vi "Material-ConfigDialog-UI.vi"(11 "error in":errorcluster) -> (15 "error out":errorcluster)   [LabVIEW 2013, in "Material-ConfigDialog.lvclass"]
uses:
  Material-ConfigDialog.lvclass
  Reuse Library/featherweight/Core/Sequencer/FTW-Sequencer.lvclass/FTW-Sequencer.ctl
  Material-ConfigDialog-Page.ctl
  Reuse Library/featherweight/Core/Messaging/Messenger.Actor/FTW-Messenger-Actor.lvclass
  <instrlib>/Keyence LK-G5000/Public/Constant/Comm Interface.ctl
  Glue/Material-Glue-TreeItem.ctl
  Reuse Library/featherweight/Core/Regex/FTW-Regex.vi
  Reuse Library/featherweight/Core/Error/FTW-ERR-StatusException.vi
  Reuse Library/featherweight/Core/Error/FTW-ERR-Clear.vi
  Reuse Library/featherweight/Core/Error/FTW-ERR-ThrowError.vi
  Deploy Application/Material-Application-Constants.vi
  Reuse Library/featherweight/Core/Sequencer/FTW-Sequencer.lvclass
  Reuse Library/featherweight/Core/Messaging/Message.Actor/FTW-Message-Actor.lvclass
  Automation/Material-Automation-Website.ctl
  <instrlib>/Keyence LK-G5000/Keyence LK-G5000.lvlib
panel:
  in  "UI_Tree_Navigation":string(tree) caption="Navigation Tree"
  in  "Hidden Controls\n(Tab Control Container)":enum32{"Just some hidden controls"}(tab)
  out "Status Bar Messages":string
  in  "UI-Button-Save":bool caption="Save Button"
  in  "UI-Button-Cancel":bool caption="Cancel Button"
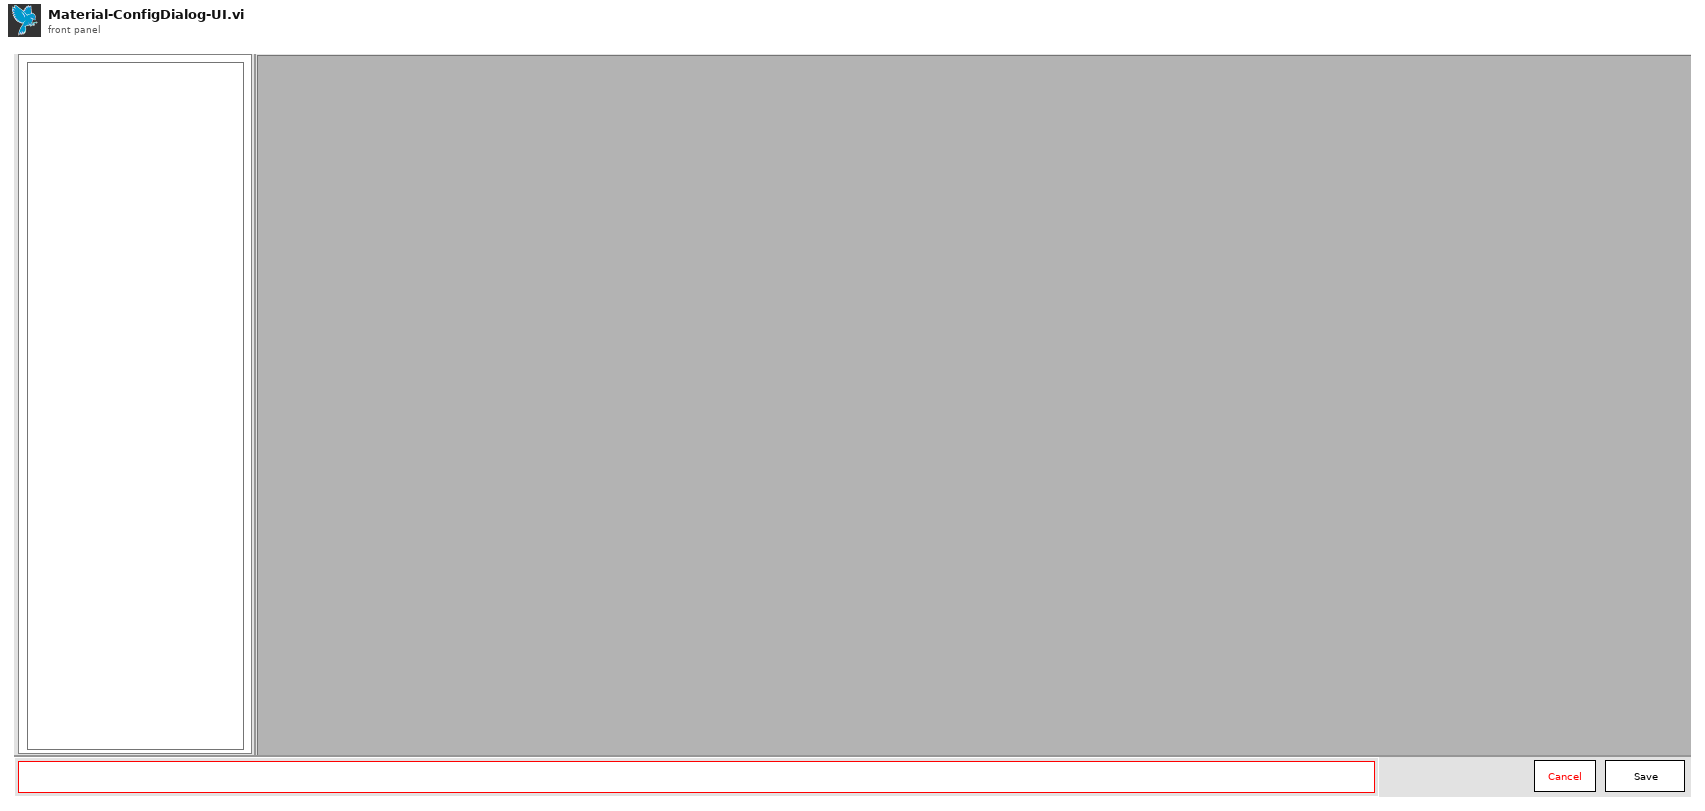
[diagram p1: front panel]
types:
  T1 = typedef "Material-Automation-Website.ctl" = enum16{"Wirebird Labs Home", "Wirebird Labs Support Home", "Wirebird Labs Licensing", "Wirebird Labs Idea Exchange", "Wirebird Labs Report a Bug", "Wirebird Labs Services Status", "Contact Wirebird Labs", "Deploy Documentation", "Deploy Credits", "Deploy Marketing", "Deploy Feature Matrix", "Deploy Purchase", "Deploy Deployment Servers"}
  T2 = typedef "Keyence LK-G5000.lvlib/Comm Interface.ctl" = enum8{"USB", "ETHERNET"}
  T3 = typedef "Material-Glue-TreeItem.ctl" = cluster{"Tag":string, "Parent":string, "Add to Top of Parent":bool, "Type":string, "Indent":i32, "Child Only":bool, "First Cell":string, "Next Cells":string[]}
  T4 = typedef "Material-ConfigDialog.lvclass/Material-ConfigDialog-Page.ctl" = cluster{"Initialized?":bool, "PageID":string, "Messenger":refnum<class "FTW-Messenger-Actor.lvclass">}
  T5 = cluster{"Configuration Dialog Mailbox":refnum<event-registration>}
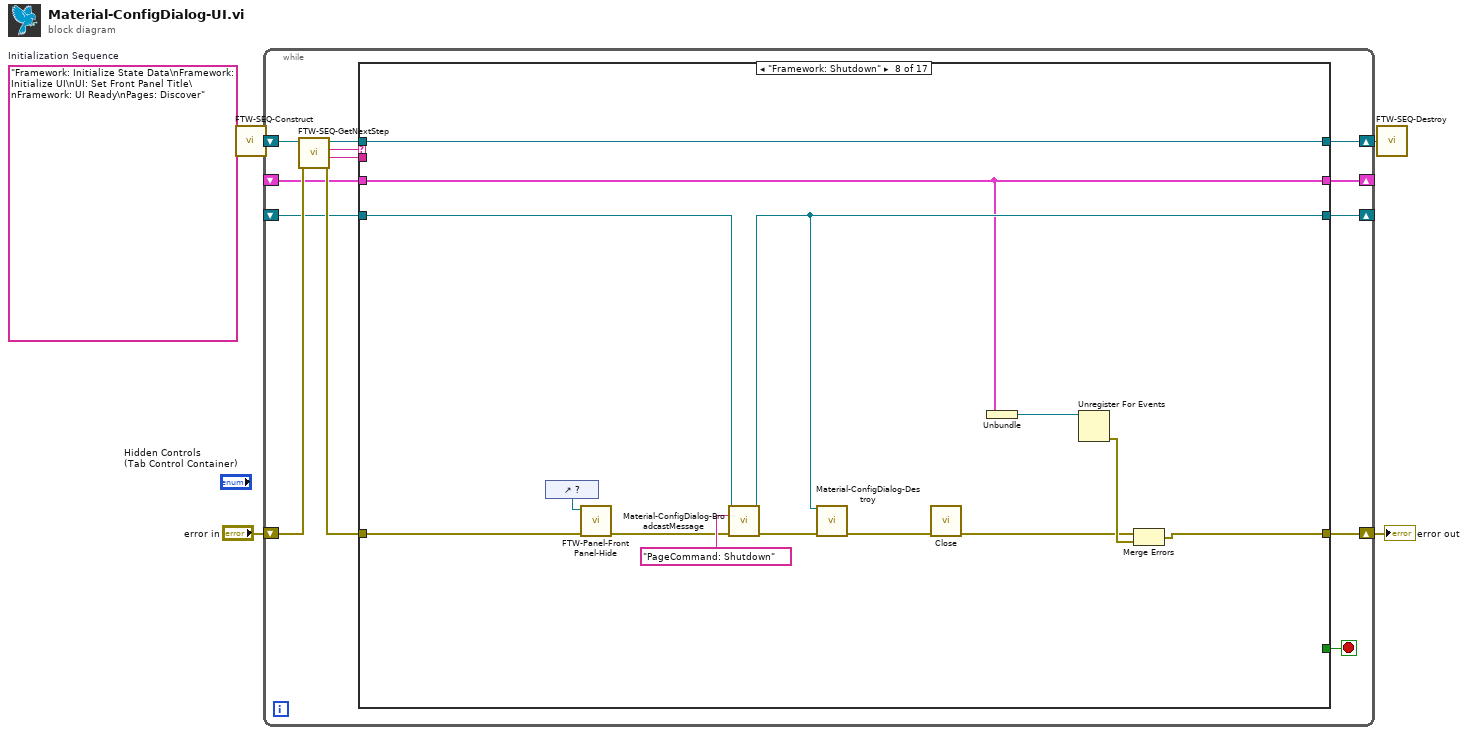
[diagram p0: block diagram]
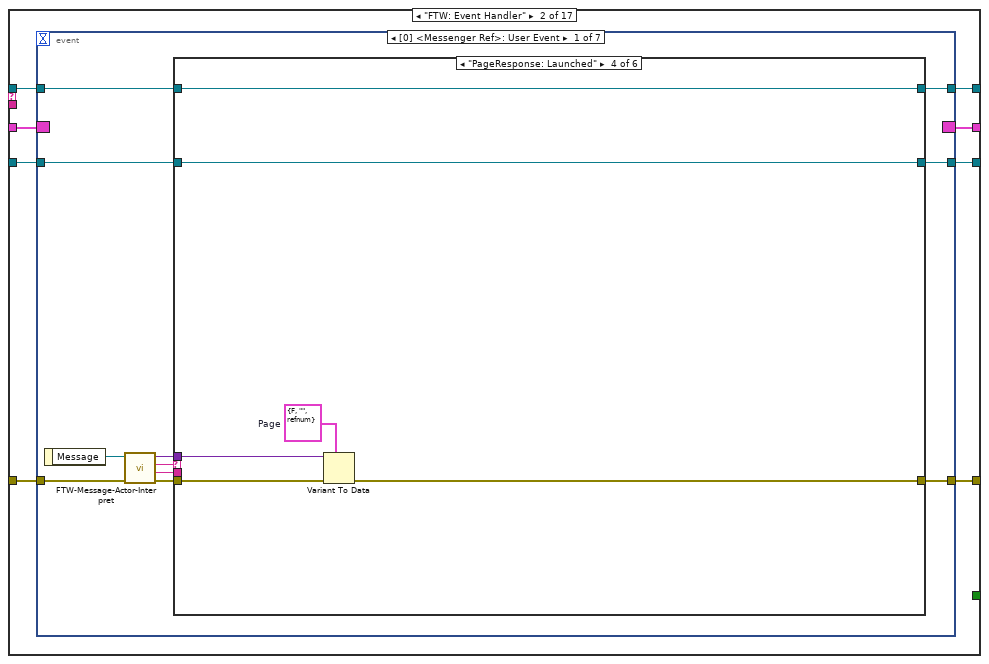
[diagram p3: hidden frame]
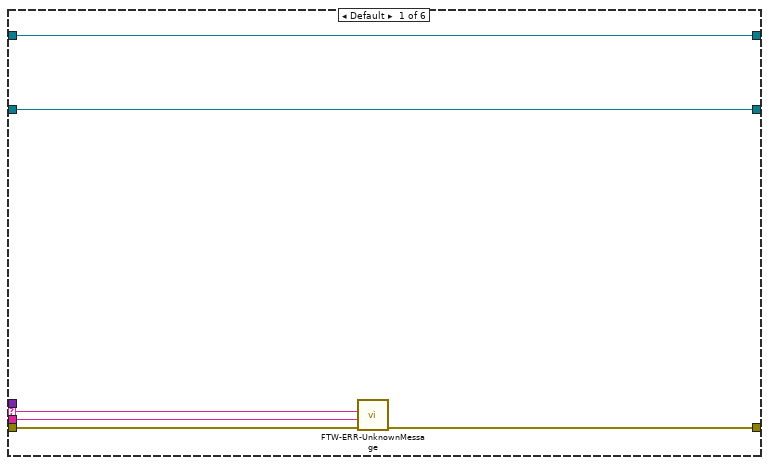
[diagram p4: hidden frame]
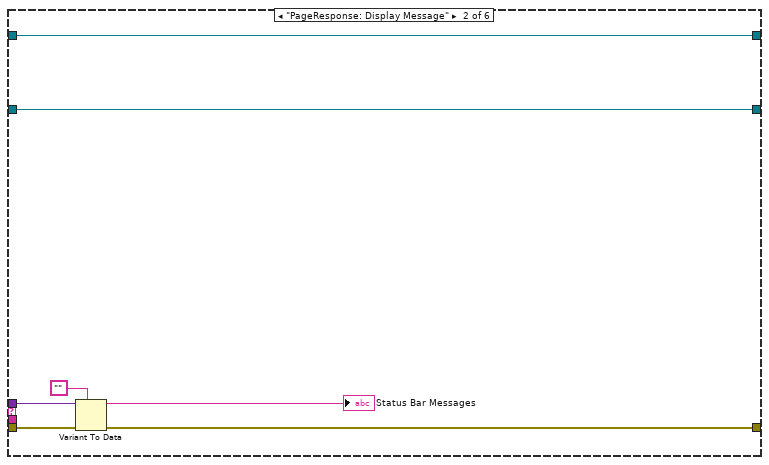
[diagram p5: hidden frame]
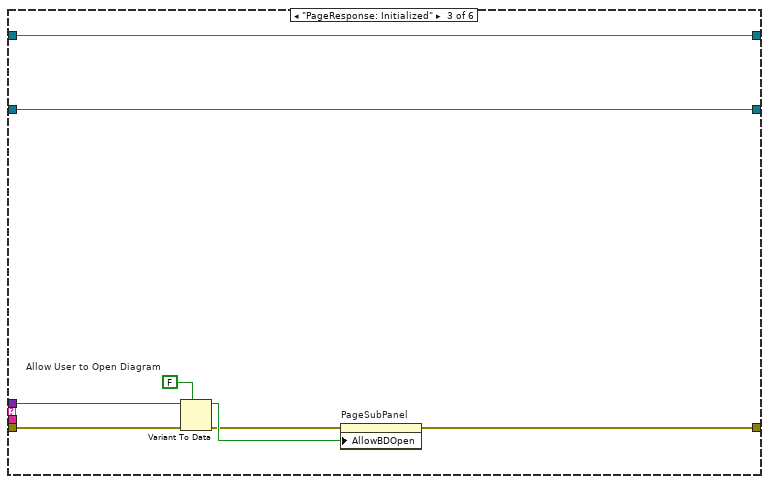
[diagram p6: hidden frame]
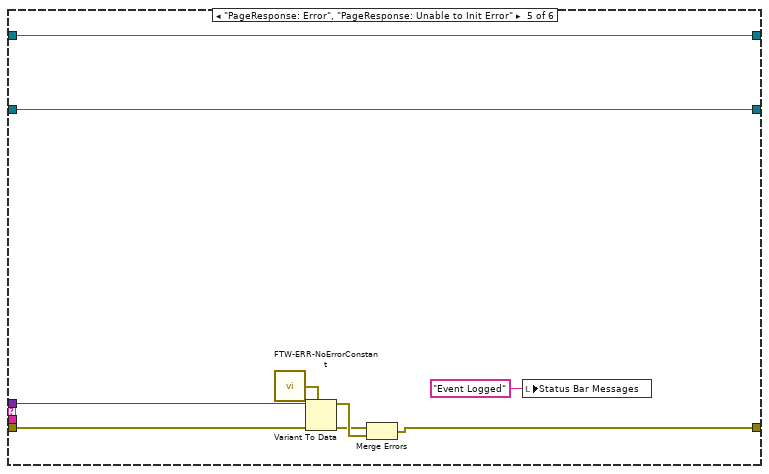
[diagram p7: hidden frame]
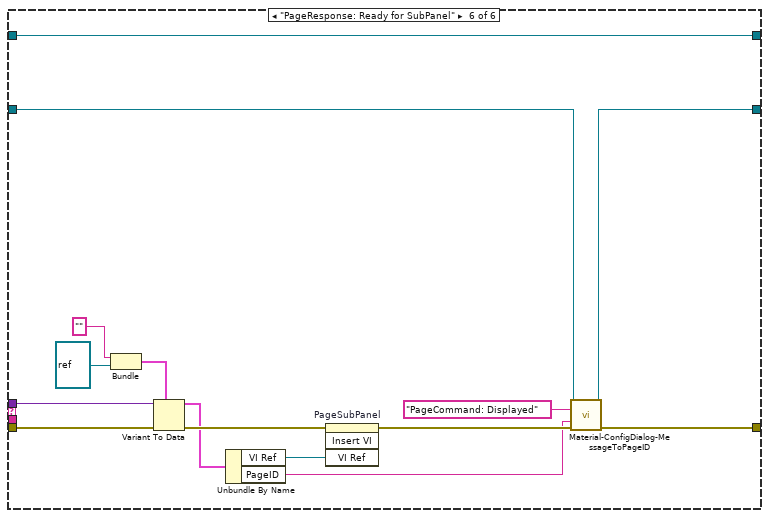
[diagram p8: hidden frame]
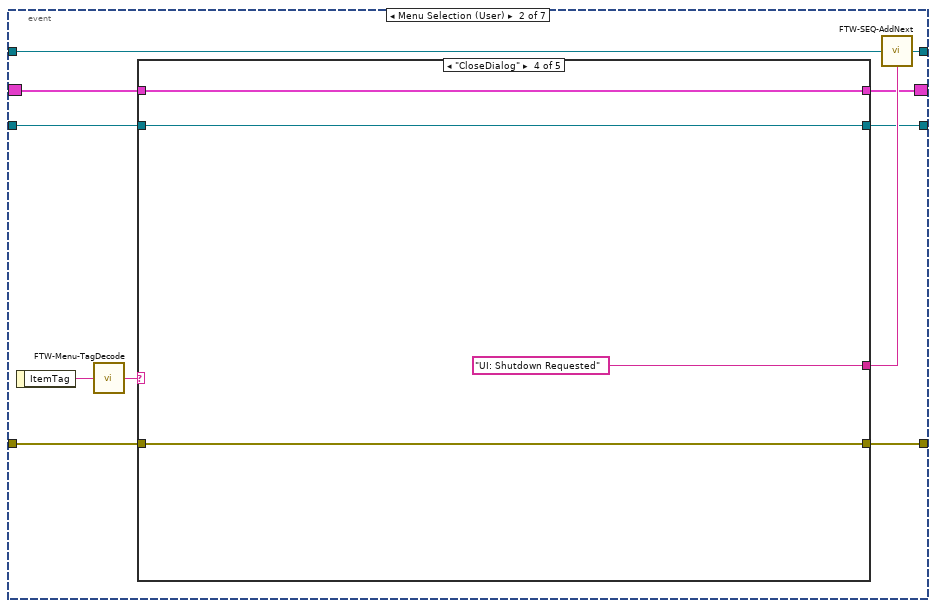
[diagram p9: hidden frame]
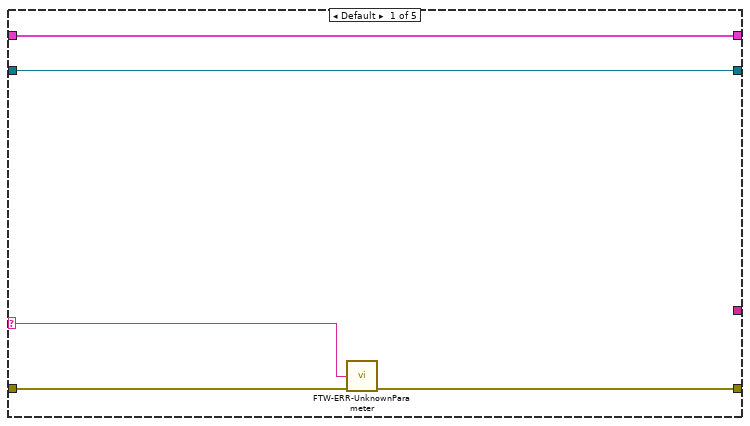
[diagram p10: hidden frame]
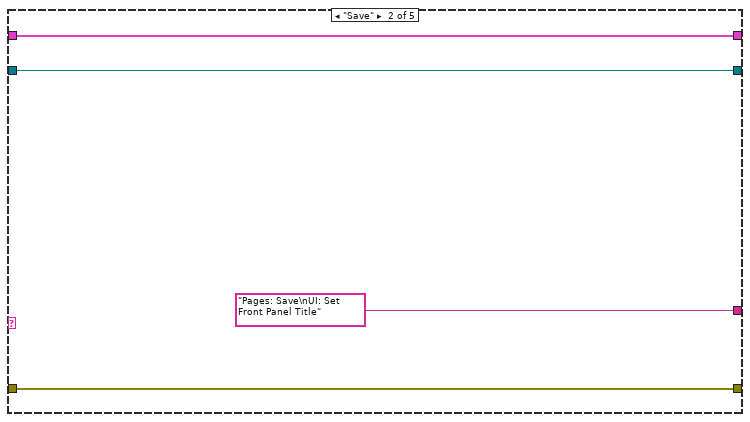
[diagram p11: hidden frame]
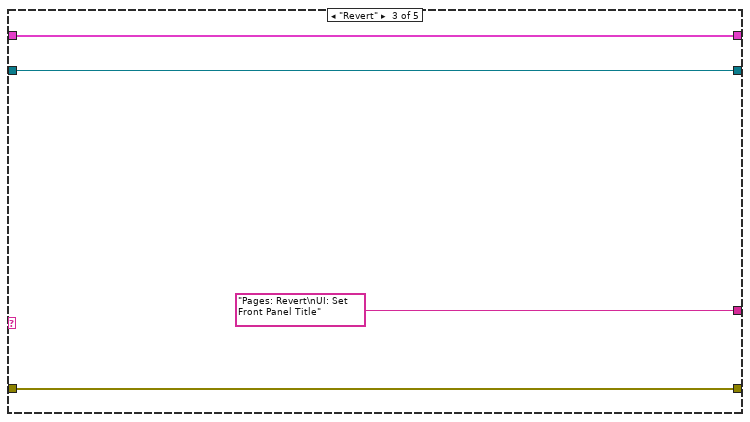
[diagram p12: hidden frame]
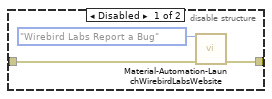
[diagram p14: hidden frame]
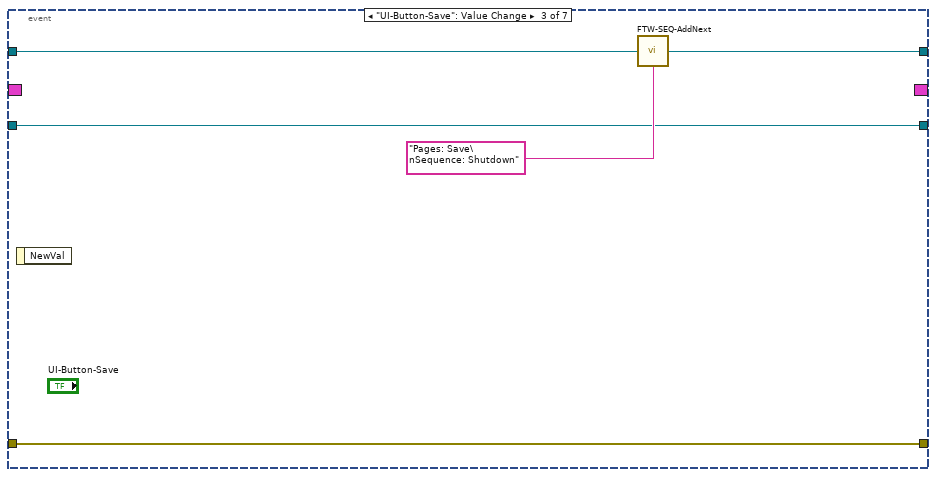
[diagram p15: hidden frame]
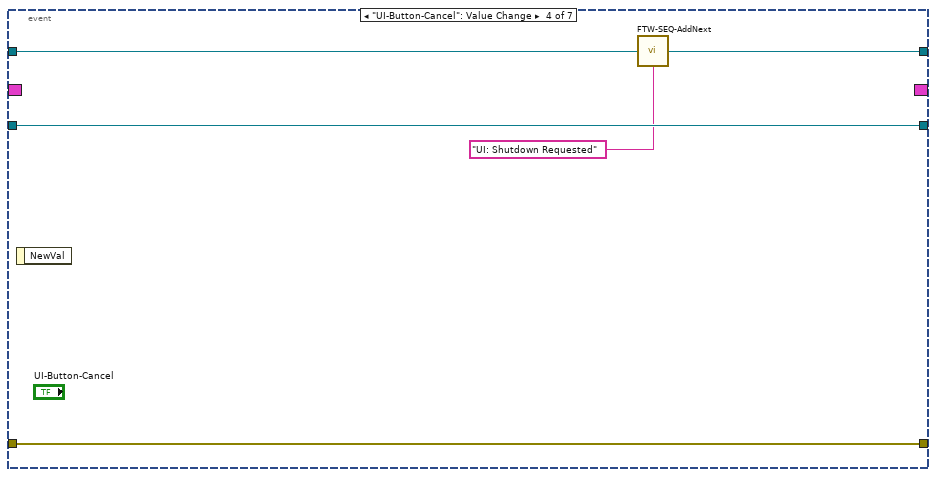
[diagram p16: hidden frame]
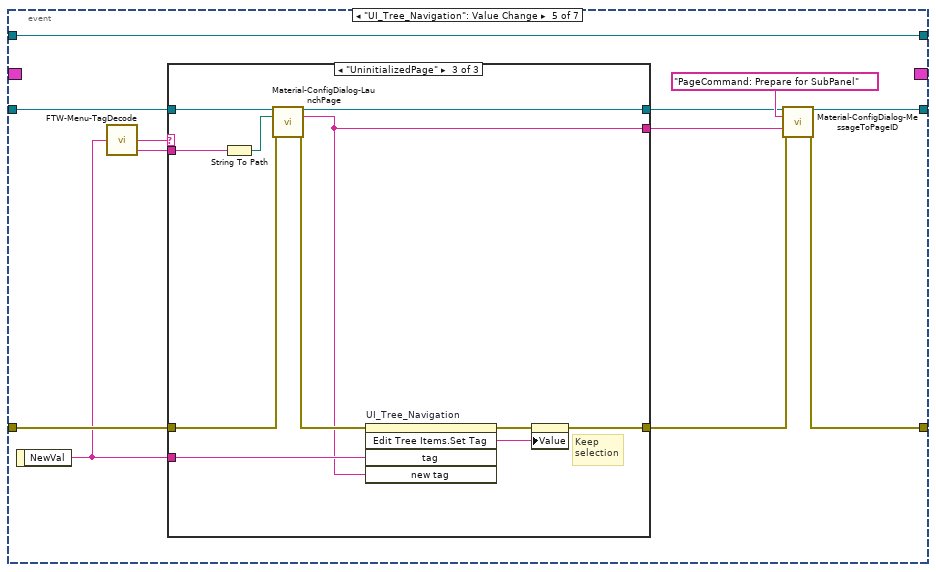
[diagram p17: hidden frame]
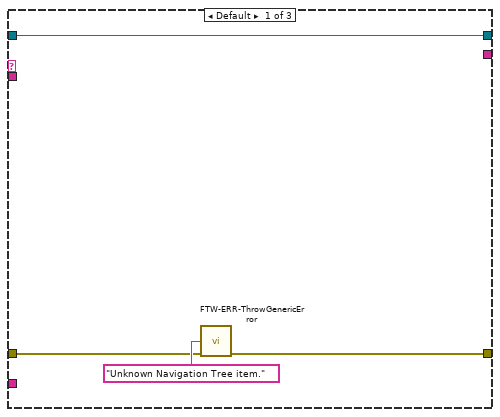
[diagram p18: hidden frame]
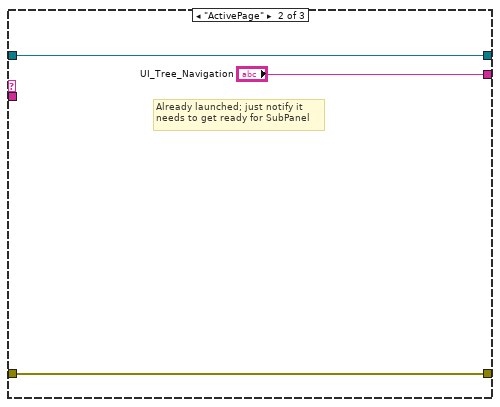
[diagram p19: hidden frame]
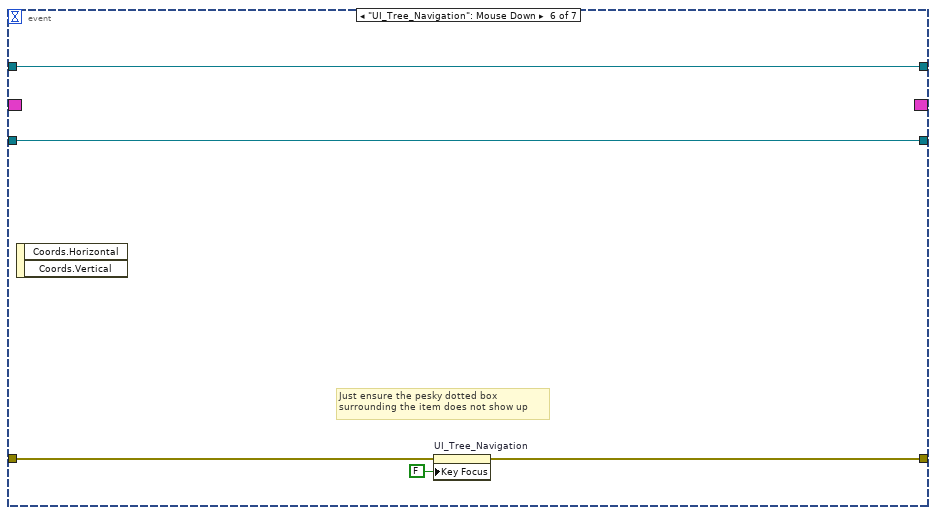
[diagram p20: hidden frame]
diagram:
  w5 = "Framework: Initialize State Data\nFramework: Initialize UI\nUI: Set Front Panel Title\nFramework: UI Ready\nPages: Discover"  # Initialization Sequence
  n1 = call "FTW-SEQ-Construct.vi"("Initial Sequence"=w5) -> ("Sequencer"=w2:refnum<class "FTW-Sequencer.lvclass">)
  n2 = while {
    shift-right: [w16] -> w1
    shift-left: w2 -> [w7]
    shift-right: [w17] -> w4
    shift-left: "error in" -> [w15]
    shift-right: [w10] -> _
    shift-left: _ -> [w11]
    shift-right: [w9] -> _
    shift-left: _ -> [w8]
    stop <- w12 stop-if-true
    n3 = call "FTW-SEQ-GetNextStep.vi"("error in"=w15, "Sequencer"=w7) -> ("error out"=w18:errorcluster, "Job Data"=w6:string, "Current Job"=w13:string, "Sequencer out"=w14:refnum<class "FTW-Sequencer.lvclass">)  [unwired: 6 in]
    n4 = case shown="\"Framework: Shutdown\"" w13 {
      selector: w13 -> [_ _ _ _ _ _ w234 _ _ _ _ _ _ _ _ _ _]
      tunnel: [w20 w28 w180 w198 w223 w229 w236 w253 w254 w262 w268 w273 w275 w291 w312 w325 w334] -> w17
      tunnel: w18 -> [w20 w27 w185 w199 w224 w230 w237 w246 w255 w262 w268 w273 w275 w291 w300 w321 w329]
      tunnel: w14 -> [w22 w30 w184 w221 w227 w233 w239 w251 w260 w264 w265 w272 w279 w293 w315 w328 w336]
      tunnel: [w22 w29 w184 w221 w227 w233 w239 w251 w260 w264 w270 w272 w281 w293 w315 w328 w336] -> w16
      tunnel: [_ _ _ _ _ _ _ _ TRUE _ _ _ _ _ _ _ _] -> w12
      tunnel: w11 -> [w21 w25 _ w220 w226 w232 w238 w243 w258 w263 w269 w274 w282 w298 w314 w327 w335]
      tunnel: [w21 w26 w186 w220 w226 w232 w238 w243 w258 w263 w269 w274 w282 w298 w314 w327 w335] -> w10
      tunnel: [w19 w24 w183 w219 w225 w231 w235 w247 w257 w261 w266 w271 w280 w294 w301 w326 w333] -> w9
      tunnel: w8 -> [w19 w23 _ w219 w225 w231 w235 w248 w257 w261 w266 w271 w280 w294 w301 w322 w330]
      tunnel: w6 -> [_ _ _ _ _ _ _ _ _ _ _ _ _ _ _ _ _]
      frame "--------- Framework ---------" {
      }
      frame "FTW: Event Handler" {
        n5 = event shown="[0] <Messenger Ref>: User Event" {
          selector: w25 -> [_ w93 _ _ _ _ _]
          dyn-events: [_ w94 _ _ _ _ _] -> w26
          timeout: _ -> [_ _ _ _ _ _ _]
          tunnel: w30 -> [w34 w99 w129 w135 w148 w170 w174]
          tunnel: [w35 w103 w133 w138 w148 w170 w177] -> w29
          tunnel: [w38 w100 w132 w136 w149 w171 w178] -> w28
          tunnel: w27 -> [w39 w101 w132 w136 w145 w172 w178]
          tunnel: [w37 w96 w130 w137 w147 w169 w175] -> w24
          tunnel: w23 -> [w36 w95 w130 w137 w142 w169 w175]
          event User Event {
            n6 = event-data() -> ("Message"=w40:refnum<class "FTW-Message.lvclass">)  [unwired: 1 in]
            n7 = call "FTW-Message-Actor-Interpret.vi"("error in"=w39, "Message"=w40) -> ("error out"=w41:errorcluster, "Sender"=w31:string, "Parameter"=w33:string, "Payload"=w32:variant)  [unwired: 6 in]
            n8 = case shown="\"PageResponse: Launched\"" w33 {
              selector: w33 -> [w43 _ _ _ _ _]
              tunnel: w32 -> [_ w54 w55 w65 w77 w92]
              tunnel: [w46 w52 w56 w63 w69 w85] -> w38
              tunnel: w41 -> [w47 w53 w60 w64 w76 w91]
              tunnel: [w44 w48 w62 w68 w73 w87] -> w37
              tunnel: w36 -> [w44 w48 w62 w68 w73 w88]
              tunnel: [w45 w49 w61 w67 w74 w90] -> w35
              tunnel: w34 -> [w45 w49 w61 w67 w74 w90]
              tunnel: w31 -> [w42 _ _ _ _ _]
              frame Default {
                n9 = call "FTW-ERR-UnknownMessage.vi"("error in"=w47, "Sender"=w42, "Unknown Parameter"=w43) -> ("error out"=w46:errorcluster)  [unwired: 8 in]
              }
              frame "PageResponse: Display Message" {
                n10 = Variant To Data(error in=w53, type="", Variant=w54) -> (data=→"Status Bar Messages":string, error out=w52:errorcluster)
              }
              frame "PageResponse: Initialized" {
                w59 = FALSE  # Allow User to Open Diagram
                n11 = Variant To Data(error in=w60, type=w59, Variant=w55) -> (data=w58:bool, error out=w57:errorcluster)
                n12 = property on="PageSubPanel" class="SubPnl"(error in=w57, "AllowBDOpen"=w58) -> (error out=w56:errorcluster)  [unwired: 1 in, 1 out]
              }
              frame "PageResponse: Launched" {
                w66 = T4 {"Initialized?"=FALSE, "PageID"="", "Messenger"=refnum}  # Page
                n13 = Variant To Data(error in=w64, type=w66, Variant=w65) -> (error out=w63:errorcluster)  [unwired: 1 out]
              }
              frame "PageResponse: Error", "PageResponse: Unable to Init Error" {
                n14 = call "FTW-ERR-NoErrorConstant.vi"() -> ("no error"=w75:errorcluster)
                n15 = Variant To Data(error in=w76, type=w75, Variant=w77) -> (data=w71:errorcluster, error out=w70:errorcluster)
                n16 = Merge Errors(w70, w71) -> (w69:errorcluster)
                n17 = local write "Status Bar Messages"("Event Logged" ("Status Bar Messages")) -> ()
              }
              frame "PageResponse: Ready for SubPanel" {
                n18 = Bundle("PageID"="", "VI Ref"=refnum<vi> refnum) -> (w81:cluster{"PageID":string, "VI Ref":refnum<vi>})  [unwired: 1 in]
                n19 = Variant To Data(error in=w91, type=w81, Variant=w92) -> (data=w80:cluster{"PageID":string, "VI Ref":refnum<vi>}, error out=w84:errorcluster)
                n20 = Unbundle By Name(w80) -> ("VI Ref"=w79:refnum<vi>, "PageID"=w78:string)
                n21 = invoke on="PageSubPanel" class="SubPanel" method="Insert VI"(error in=w84, "VI Ref"=w79) -> (error out=w86:errorcluster)  [unwired: 2 in, 3 out]
                n22 = call "Material-ConfigDialog-MessageToPageID.vi"("Configuration Dialog"=w88, "Parameter"="PageCommand: Displayed", "PageID"=w78, "error in"=w86) -> ("Configuration Dialog out"=w87:refnum<class "Material-ConfigDialog.lvclass">, "error out"=w85:errorcluster)  [unwired: 10 in]
              }
            }
          }
          event Menu Selection (User) {
            n23 = event-data() -> ("ItemTag"=w98:string)  [unwired: 1 in]
            n24 = call "FTW-Menu-TagDecode.vi"("Menu Item Tag"=w98) -> ("Command"=w97:string)  [unwired: 1 in, 2 out]
            n25 = case shown="\"CloseDialog\"" w97 {
              selector: w97 -> [w105 _ _ _ _]
              tunnel: [_ "Pages: Save\nUI: Set Front Panel Title" ("Add to Top of Queue") "Pages: Revert\nUI: Set Front Panel Title" ("Add to Top of Queue") "UI: Shutdown Requested" ("Add to Top of Queue") _] -> w102
              tunnel: w101 -> [w108 w111 w115 w119 w124]
              tunnel: [w107 w111 w115 w119 w123] -> w100
              tunnel: [w106 w110 w114 w118 w122] -> w96
              tunnel: w95 -> [w106 w110 w114 w118 w122]
              tunnel: [w104 w109 w113 w117 w121] -> w94
              tunnel: w93 -> [w104 w109 w113 w117 w121]
              frame Default {
                n26 = call "FTW-ERR-UnknownParameter.vi"("Unknown Parameter"=w105, "error in"=w108) -> ("error out"=w107:errorcluster)  [unwired: 13 in]
              }
              frame "Save" {
              }
              frame "Revert" {
              }
              frame "CloseDialog" {
              }
              frame "ReportBug" {
                n27 = disable-structure shown="Enabled" {
                  disable-tunnel: w124 -> [w127 w128]
                  disable-tunnel: [w126 w128] -> w123
                  frame Disabled {
                    n28 = call "Material-Automation-LaunchWirebirdLabsWebsite.vi"("Site to Launch"=Material-Automation-Website."Wirebird Labs Report a Bug", "error in"=w127) -> ("error out"=w126:errorcluster)  [unwired: 13 in]
                  }
                  frame Enabled {
                  }
                }
              }
            }
            n29 = call "FTW-SEQ-AddNext.vi"("Add Next in Sequence"=w102, "Sequencer"=w99) -> ("Sequencer out"=w103:refnum<class "FTW-Sequencer.lvclass">)  [unwired: 2 in]
          }
          event "UI-Button-Save": Value Change {
            n30 = event-data() -> ()  [unwired: 1 in, 1 out]
            n31 = call "FTW-SEQ-AddNext.vi"("Add Next in Sequence"="Pages: Save\nSequence: Shutdown" ("Add to Top of Queue"), "Sequencer"=w129) -> ("Sequencer out"=w133:refnum<class "FTW-Sequencer.lvclass">)  [unwired: 2 in]
          }
          event "UI-Button-Cancel": Value Change {
            n32 = event-data() -> ()  [unwired: 1 in, 1 out]
            n33 = call "FTW-SEQ-AddNext.vi"("Add Next in Sequence"="UI: Shutdown Requested" ("Add to Top of Queue"), "Sequencer"=w135) -> ("Sequencer out"=w138:refnum<class "FTW-Sequencer.lvclass">)  [unwired: 2 in]
          }
          event "UI_Tree_Navigation": Value Change {
            n34 = event-data() -> ("NewVal"=w140:string)  [unwired: 1 in]
            n35 = call "FTW-Menu-TagDecode.vi"("Menu Item Tag"=w140) -> ("Command"=w146:string, "Payload"=w143:string)  [unwired: 1 in, 1 out]
            n36 = case shown="\"UninitializedPage\"" w146 {
              tunnel: w145 -> [w153 w157 w168]
              tunnel: [w152 w157 w159] -> w144
              tunnel: w143 -> [_ _ w167]
              tunnel: w142 -> [w151 w156 w165]
              tunnel: [w151 w156 w164] -> w141
              tunnel: w140 -> [_ _ w162]
              tunnel: [_ "UI_Tree_Navigation" w161] -> w139
              frame Default {
                n37 = call "FTW-ERR-ThrowGenericError.vi"("Error Message"="Unknown Navigation Tree item.", "error in"=w153) -> ("error out"=w152:errorcluster)  [unwired: 13 in]
              }
              frame "ActivePage" {
                # "Already launched; just notify it\nneeds to get ready for SubPanel"
              }
              frame "UninitializedPage" {
                # "Keep\nselection"
                n38 = String To Path(string=w167) -> (path=w166:path)
                n39 = call "Material-ConfigDialog-LaunchPage.vi"("Configuration Dialog"=w165, "Configuration Page VI Filepath"=w166, "error in"=w168) -> ("Configuration Dialog out"=w164:refnum<class "Material-ConfigDialog.lvclass">, "New Navigation Tree Tag"=w161:string, "error out"=w163:errorcluster)  [unwired: 9 in, 1 out]
                n40 = invoke on="UI_Tree_Navigation" class="Tree (strict)" method="Edit Tree Items.Set Tag"(error in=w163, "tag"=w162, "new tag"=w161) -> (error out=w160:errorcluster, "Edit Tree Items:Set Tag"=w158:string)  [unwired: 2 in, 3 out]
                n41 = property on="UI_Tree_Navigation" class="Tree (strict)"(error in=w160, "Value"=w158) -> (error out=w159:errorcluster)  [unwired: 1 in, 1 out]
              }
            }
            n42 = call "Material-ConfigDialog-MessageToPageID.vi"("Configuration Dialog"=w141, "Parameter"="PageCommand: Prepare for SubPanel", "PageID"=w139, "error in"=w144) -> ("Configuration Dialog out"=w147:refnum<class "Material-ConfigDialog.lvclass">, "error out"=w149:errorcluster)  [unwired: 10 in]
          }
          event "UI_Tree_Navigation": Mouse Down {
            # "Just ensure the pesky dotted box\nsurrounding the item does not show up"
            n43 = event-data() -> ()  [unwired: 1 in, 2 out]
            n44 = property on="UI_Tree_Navigation" class="Tree (strict)"(error in=w172, "Key Focus"=FALSE) -> (error out=w171:errorcluster)  [unwired: 1 in, 1 out]
          }
          event Panel Close? {
            n45 = event-data() -> ()  [unwired: 1 in, 1 out]
            n46 = call "FTW-SEQ-AddNext.vi"("Add Next in Sequence"="UI: Shutdown Requested" ("Add to Top of Queue"), "Sequencer"=w174) -> ("Sequencer out"=w177:refnum<class "FTW-Sequencer.lvclass">)  [unwired: 2 in]
            n47 = event-data("Discard?"=TRUE) -> ()  [unwired: 1 in, 1 out]
          }
        }
      }
      frame "Framework: Initialize State Data" {
        n48 = call "Material-ConfigDialog-Construct.vi"("error in"=w185) -> ("Configuration Dialog"=w183:refnum<class "Material-ConfigDialog.lvclass">, "Configuration Dialog Mailbox"=w187:refnum<event-registration>, "error out"=w181:errorcluster)  [unwired: 12 in]
        n49 = call <instrlib>:"Initialize.vi"("error in (no error)"=w181, "Comm Interface"=Comm_Interface."USB") -> ("error out"=w180:errorcluster)  [unwired: 9 in]
        n50 = Bundle("Configuration Dialog Mailbox"=w187) -> (w186:T5)  [unwired: 1 in]
      }
      frame "Framework: Initialize UI" {
        w195 = cluster{"Height":i16, "Width":i16} {"Height"=2, "Width"=2}  # Breathing Room
        w201 = i16 40 ("Vertical")
        w204 = i16 240 ("Horizontal")
        w211 = 2000  # Much wider than ever expected to be
        n51 = invoke on="UI_Tree_Navigation" class="Tree (strict)" method="Edit Tree Items.Delete"("Delete Children"=TRUE ("Delete Children?")) -> (error out=w193:errorcluster)  [unwired: 4 in, 4 out]
        n52 = call "Material-Application-MinimumPageSize.vi"("error in"=w199) -> ("Minimum Pane Size"=w192:cluster{"Horizontal":i16, "Vertical":i16}, "error out"=w210:errorcluster)  [unwired: 13 in]
        n53 = Bundle By Name(cluster=w192, "Horizontal"=w204) -> (w209:cluster{"Horizontal":i16, "Vertical":i16})
        n54 = Bundle By Name(cluster=w192, "Horizontal"=i16 310, "Vertical"=w201) -> (w208:cluster{"Horizontal":i16, "Vertical":i16})
        n55 = global read "Material-Application-Constants.vi" "Color.Selection"() -> (w189:u32)
        n56 = Add(x=cluster{"Horizontal":i16, "Vertical":i16} {"Horizontal"=24, "Vertical"=0}, y=w192) -> (x+y=w190:cluster{"Horizontal":i16, "Vertical":i16})
        n57 = Unbundle By Name(w190) -> ("Horizontal"=w205:i16, "Vertical"=w202:i16)
        n58 = property on="UserInterface-Pane-Page" class="Pane"(error in=w210, "Minimum Pane Size"=w190) -> (error out=w217:errorcluster)  [unwired: 1 in, 1 out]
        n59 = property on="UserInterface-Pane-Navigation" class="Pane"("Minimum Pane Size"=w209) -> (error out=w215:errorcluster)  [unwired: 2 in, 1 out]
        n60 = property on="UserInterface-Pane-Buttons" class="Pane"("Minimum Pane Size"=w208) -> (error out=w214:errorcluster)  [unwired: 2 in, 1 out]
        n61 = property on="UI_Tree_Navigation" class="Tree (strict)"(error in=w193, "Value"="", "SelMode"=1 ("Selection Mode"), "ActiveColNum"=0 ("Active Cell:Active Column Number"), "Width"=w211, "SelColor"=w189) -> (error out=w188:errorcluster)  [unwired: 1 in, 1 out]
        n62 = Add(x=w204, y=w205) -> (x+y=w203:i16)
        n63 = Add(x=w201, y=w202) -> (x+y=w200:i16)
        n64 = Bundle By Name(cluster=cluster{"Height":i16, "Width":i16} {"Height"=0, "Width"=0} ("Size"), "Height"=w200, "Width"=w203) -> (w206:cluster{"Height":i16, "Width":i16})
        n65 = Merge Errors(w188, w217, w215, w214) -> (w216:errorcluster)
        n66 = Add(x=w195, y=w206) -> (x+y=w196:cluster{"Height":i16, "Width":i16})
        n67 = invoke class="VI" method="FP.Run-Time Position.Centered"(error in=w216, "Monitor"=w196) -> (error out=w198:errorcluster)  [unwired: 3 in, 4 out]
      }
      frame "Framework: UI Ready" {
        n68 = control-ref of="?"() -> (w222:refnum<vi>)
        n69 = call "FTW-Panel-FrontPanel-Open.vi"("error in"=w224, "VI Ref"=w222) -> ("error out"=w223:errorcluster)  [unwired: 8 in, 1 out]
      }
      frame "FTW: Error Handler" {
        n70 = call "FTW-ERR-SerializeForLog.vi"("error in"=w230) -> ("Serialized Error"=w228:string)
        n71 = local write "Status Bar Messages"(w228) -> ()
        n72 = call "FTW-ERR-NoErrorConstant.vi"() -> ("no error"=w229:errorcluster)
      }
      frame "FTW: Unknown Job", Default {
        n73 = call "FTW-ERR-UnknownJob.vi"("error in"=w237, "Unknown Job"=w234) -> ("error out"=w236:errorcluster)  [unwired: 9 in]
      }
      frame "Framework: Shutdown" {
        n74 = control-ref of="?"() -> (w244:refnum<vi>)
        n75 = call "FTW-Panel-FrontPanel-Hide.vi"("error in"=w246, "VI Ref"=w244) -> ("error out"=w245:errorcluster)  [unwired: 8 in, 1 out]
        n76 = call "Material-ConfigDialog-BroadcastMessage.vi"("Configuration Dialog"=w248, "Parameter"="PageCommand: Shutdown", "error in"=w245) -> ("Configuration Dialog out"=w247:refnum<class "Material-ConfigDialog.lvclass">, "error out"=w249:errorcluster)  [unwired: 11 in]
        n77 = call "Material-ConfigDialog-Destroy.vi"("Configuration Dialog"=w247, "error in"=w249) -> ("error out"=w241:errorcluster)  [unwired: 13 in]
        n78 = call <instrlib>:"Close.vi"("error in (no error)"=w241) -> ("error out"=w240:errorcluster)  [unwired: 10 in]
        n79 = Unbundle(w243) -> ("Configuration Dialog Mailbox"=w242:refnum<event-registration>)
        n80 = Unregister For Events(event registration refnum=w242) -> (error out=w252:errorcluster)  [unwired: 1 in]
        n81 = Merge Errors(w240, w252) -> (w253:errorcluster)
      }
      frame "Framework: Exit" {
        n82 = control-ref of="?"() -> (w256:refnum<vi>)
        n83 = call "FTW-Panel-FrontPanel-Close.vi"("error in"=w255, "VI Ref"=w256) -> ("error out"=w254:errorcluster)  [unwired: 8 in, 1 out]
      }
      frame "--------- Sequences ---------" {
      }
      frame "Sequence: Shutdown" {
        w267 = "Framework: Shutdown\nFramework: Exit"  # Application Shutdown
        n84 = call "FTW-SEQ-AddNext.vi"("Add Next in Sequence"=w267, "Sequencer"=w265) -> ("Sequencer out"=w270:refnum<class "FTW-Sequencer.lvclass">)  [unwired: 2 in]
      }
      frame "--------- Application Logic ---------" {
      }
      frame "UI: Shutdown Requested" {
        w276 = TRUE  # Shutdown Conditionally Allowed?
        n85 = case shown="True" w276 {
          tunnel: [w283 w287] -> w278
          tunnel: "Sequence: Shutdown" ("Add to Top of Queue") -> [w283 w285]
          frame False {
          }
          frame True {
            w286 = ""  # Do nothing... return to dialog without shutting down.
            n86 = Two Button Dialog(message="Are you sure you want to shut down?", 1:"Shutdown now" ("F button name (\"Cancel\")"), 2:"Not yet" ("T button name (\"OK\")")) -> (T button?=w288:bool)
            n87 = Select(t=w286, s=w288, f=w285) -> (s? t:f=w287:string)
          }
        }
        n88 = call "FTW-SEQ-AddNext.vi"("Add Next in Sequence"=w278, "Sequencer"=w279) -> ("Sequencer out"=w281:refnum<class "FTW-Sequencer.lvclass">)  [unwired: 2 in]
      }
      frame "UI: Set Front Panel Title" {
        w292 = FALSE  # Show Dirty Dot?
        n89 = Select(t="Deployment Configuration*", s=w292, f="Deployment Configuration") -> (s? t:f=w297:string)
        n90 = property class="VI"("Front Panel.Title"=w297) -> ()  [unwired: 2 in, 2 out]
      }
      frame "Pages: Discover" {
        w305 = FALSE  # Collapse all new items?
        w308 = TRUE  # Delete Tree Items First?
        # "Make it go to the default page; in the future,\nthis can be replaced by a \"Last Page Visited\""
        n91 = call "Material-ConfigDialog-DiscoverPages.vi"("Custom Config Pages Directory"=path "", "error in"=w300) -> ("Display Names"=w303:string[], "Tree Tags"=w304:string[], "error out"=w302:errorcluster)  [unwired: 9 in, 2 out]
        n92 = for {
          tunnel: T3 {"Tag"="", "Parent"="", "Add to Top of Parent"=FALSE, "Type"="", "Indent"=0, "Child Only"=FALSE, "First Cell"="", "Next Cells"=[]} -> [w320]
          tunnel: [w319] -> w306 mode=indexing
          tunnel: w304 -> [w316] mode=indexing
          tunnel: w303 -> [w318] mode=indexing
          n93 = Bundle By Name(cluster=w320, "Child Only"=TRUE, "First Cell"=w318, "Tag"=w316) -> (w319:T3)
        }
        n94 = control-ref of="UI_Tree_Navigation"() -> (w310:refnum<vi>)
        n95 = call "Material-Glue-Tree-AddItems.vi"("Tree Ctl Ref"=w310, "Tree Items to Create"=w306, "Delete Tree Items First?"=w308, "Collapse all new items?"=w305, "error in"=w302) -> ("error out"=w309:errorcluster)  [unwired: 8 in, 2 out]
        n96 = Index Array(array=w304, index=0) -> (element=w311:string)
        n97 = property on="UI_Tree_Navigation" class="Tree (strict)"(error in=w309, "Val(Sgnl)"=w311) -> (error out=w312:errorcluster)  [unwired: 1 in, 1 out]
      }
      frame "Pages: Save" {
        n98 = local read "UI_Tree_Navigation"() -> (w324:string)
        n99 = call "Material-ConfigDialog-MessageToPageID.vi"("Configuration Dialog"=w322, "Parameter"="PageCommand: Settings Saved", "PageID"=w324, "error in"=w321) -> ("Configuration Dialog out"=w326:refnum<class "Material-ConfigDialog.lvclass">, "error out"=w325:errorcluster)  [unwired: 10 in]
      }
      frame "Pages: Revert" {
        n100 = local read "UI_Tree_Navigation"() -> (w332:string)
        n101 = call "Material-ConfigDialog-MessageToPageID.vi"("Configuration Dialog"=w330, "Parameter"="PageCommand: Revert", "PageID"=w332, "error in"=w329) -> ("Configuration Dialog out"=w333:refnum<class "Material-ConfigDialog.lvclass">, "error out"=w334:errorcluster)  [unwired: 10 in]
      }
    }
  }
  "error out" <- w4
  n102 = call "FTW-SEQ-Destroy.vi"("Sequencer"=w1) -> ()  [unwired: 1 in]
